vi "main.vi"(1 "op":string, 2 "num2":dbl, 3 "num1":dbl) -> (0 "result":dbl)   [LabVIEW 2022 SP3]
uses:
  <vilib>/wsapi/Web Request.lvclass
panel:
  in  "LabVIEW Web Service Request":refnum<class "Web Request.lvclass">
  # "Use the Web Service Request input terminal to call the VIs on the Web Services palette. Do not remove it from the connector pane unless you don't need access to the palette."
  # "Each additional control wired to the connector pane will be available as an input in the URL. To include an indicator in terminal-mode output (the default setting), it must also be wired to the connector pane."
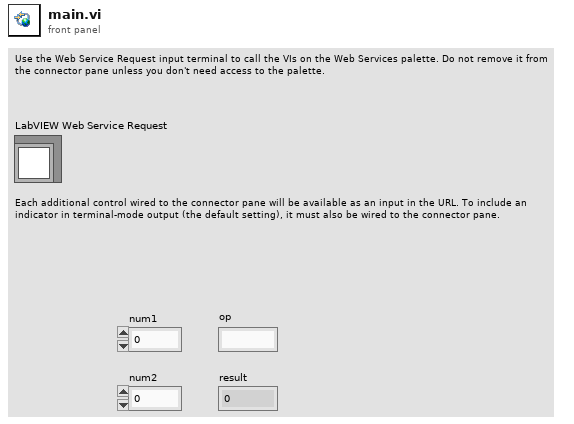
[diagram p1: front panel]
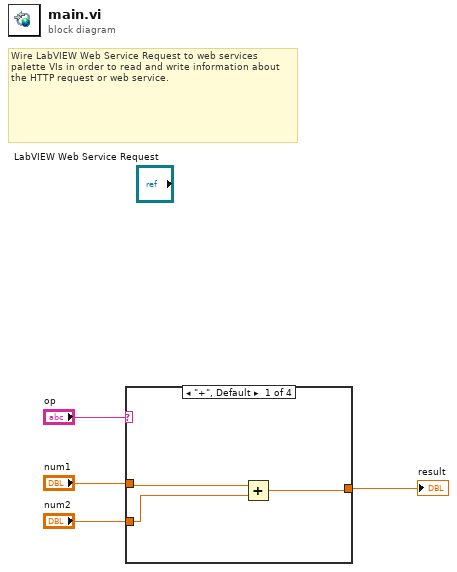
[diagram p0: block diagram]
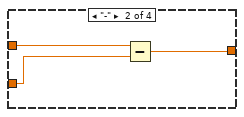
[diagram p2: hidden frame]
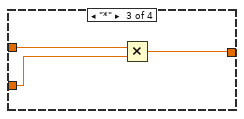
[diagram p3: hidden frame]
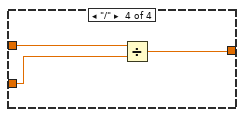
[diagram p4: hidden frame]
diagram:
  # "Wire LabVIEW Web Service Request to web services palette VIs in order to read and write information about the HTTP request or web service."
  n1 = case shown="\"+\", Default" "op" {
    tunnel: "num2" -> [w5 w9 w12 w15]
    tunnel: "num1" -> [w6 w10 w13 w16]
    tunnel: [w7 w8 w11 w14] -> w1
    frame "+", Default {
      n2 = Add(x=w6, y=w5) -> (x+y=w7:dbl)
    }
    frame "-" {
      n3 = Subtract(x=w10, y=w9) -> (x-y=w8:dbl)
    }
    frame "*" {
      n4 = Multiply(x=w13, y=w12) -> (x*y=w11:dbl)
    }
    frame "/" {
      n5 = Divide(x=w16, y=w15) -> (x/y=w14:dbl)
    }
  }
  "result" <- w1
